vi "read from FIFO.vi"(10 "Read size":u32, 11 "Refnum in":refnum<k20>) -> (0 "data read?":bool, 1 "Data":sgl[](array[numeric]), 2 "FIFO level":u32, 3 "FPGA VI Reference Out":refnum<k20>)   [LabVIEW 2018]
uses:
  <vilib>/Utility/error.llb/Error Cluster From Error Code.vi
  <vilib>/rvi/errors/niLvFpgaAdjustHostInterfaceError.vi
  <vilib>/rvi/interface/nirviMethod/nirviMethod.xnode
  <vilib>/FPGAPlugInAG/Dynamic/niLvFpga_ReadFifo_Dynamic.vi
  <vilib>/rvi/errors/niLvFpgaMergeErrorWithErrorCode.vi
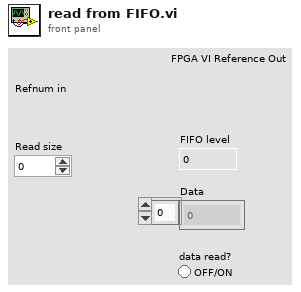
[diagram p1: front panel]
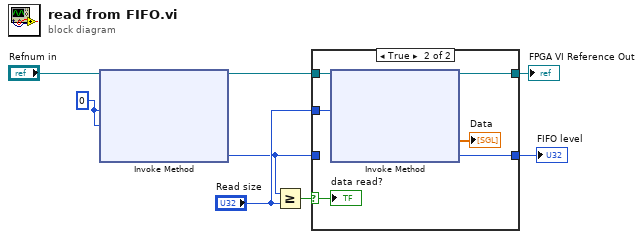
[diagram p0: block diagram]
diagram:
  w6 = u32 0 ("Number of Elements")
  n1 = xnode "Invoke Method"("FPGA VI Reference In"="Refnum in", "Number of Elements"=w6, "Timeout (ms)"=w6) -> ("FPGA VI Reference Out"=w8:refnum<k20>, "Elements Remaining"=w2:u32)  [unwired: 1 in, 2 out]
  n2 = Greater Or Equal?(x=w2, y="Read size") -> (x >= y?=w4:bool)
  n3 = case shown="True" w4 {
    selector: w4 -> [_ w13]
    tunnel: [w10 w16] -> w1
    tunnel: w8 -> [w10 w15]
    tunnel: "Read size" -> [_ w14]
    tunnel: [w9 w11] -> w3
    tunnel: w2 -> [w9 _]
    frame False {
    }
    frame True {
      n4 = xnode "Invoke Method"("FPGA VI Reference In"=w15, "Number of Elements"=w14) -> ("FPGA VI Reference Out"=w16:refnum<k20>, "Data"=→"Data":sgl[], "Elements Remaining"=w11:u32)  [unwired: 2 in, 1 out]
      "data read?" <- w13
    }
  }
  "FIFO level" <- w3
  "FPGA VI Reference Out" <- w1
